vi "BASE.SaveConfig.vi"(8 "error in (no error)":errorcluster, 10 "config file path":path, 11 "Device.Simulation in":refnum<class "Device.Simulation.lvclass">) -> (0 "error out":errorcluster, 3 "Device.Simulation out":refnum<class "Device.Simulation.lvclass">)   [LabVIEW 2019, in "Device.Simulation.lvlib" / "Device.Simulation.lvclass"]
uses:
  Device.Simulation.lvclass
  Subsystems/BASE.Device/BASE.Device/BASE.Device.lvclass
  <vilib>/Utility/config.llb/NI_LVConfig.lvlib
panel:
  out "class name":string
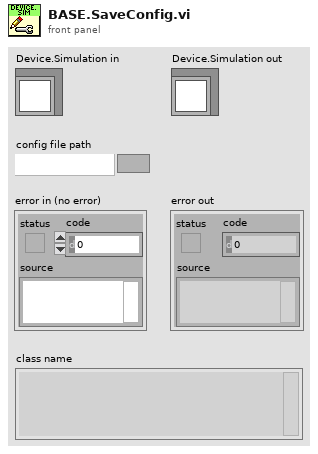
[diagram p1: front panel]
types:
  T1 = typedef "Device.Simulation.lvlib/Device.Simulation.lvclass/config--cluster.ctl" = cluster{"Name":string, "Time to Connect (ms)":u32, "Time to Check Connection (ms)":u32, "Time to Disconnect (ms)":u32, "Time to Read State (ms)":u32}
  T2 = typedef "NI_LVConfig.lvlib/Config Data RefNum.ctl" = refnum<k1>
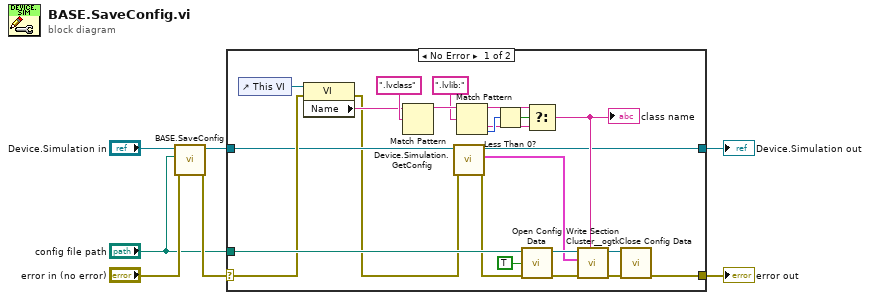
[diagram p0: block diagram]
diagram:
  n1 = call-parent "BASE.SaveConfig.vi"("error in (no error)"="error in (no error)", "config file path"="config file path", "BASE.Device in"="Device.Simulation in") -> ("error out"=w2:errorcluster, "BASE.Device out"=w5:refnum<class "Device.Simulation.lvclass">)  [unwired: 7 in]
  n2 = case shown="No Error" w2 {
    selector: w2 -> [w23 w32]
    tunnel: [w26 w32] -> w3
    tunnel: [w11 w31] -> w4
    tunnel: w5 -> [w12 w31]
    tunnel: "config file path" -> [w25 _]
    frame No Error {
      n3 = control-ref of="This VI"() -> (w24:refnum<vi>)
      n4 = property class="VI"(reference=w24, error in=w23) -> (error out=w10:errorcluster, "Name"=w14:string)  [unwired: 1 out]
      n5 = Match Pattern(string=w14, regular expression=".lvclass") -> (before substring=w20:string)  [unwired: 1 in, 3 out]
      n6 = call "Device.Simulation.GetConfig.vi"("error in (no error)"=w10, "Device.Simulation in"=w12) -> ("error out"=w9:errorcluster, "config"=w8:T1, "Device.Simulation out"=w11:refnum<class "Device.Simulation.lvclass">)  [unwired: 7 in]
      n7 = Match Pattern(string=w20, regular expression=".lvlib:") -> (before substring=w18:string, after substring=w17:string, offset past match=w21:i32)  [unwired: 1 in, 1 out]
      n8 = Less Than 0?(x=w21) -> (x < 0?=w19:bool)
      n9 = call <vilib>:"Open Config Data.vi"("error in (no error)"=w9, "create file if necessary (T)"=TRUE, "configuration file path"=w25) -> ("error out"=w29:errorcluster, "refnum"=w30:T2)  [unwired: 6 in, 1 out]
      n10 = Select(t=w18, s=w19, f=w17) -> (s? t:f=w13:string)
      "class name" <- w13
      n11 = call <userlib>:"Write Section Cluster__ogtk.vi"("section (optional)"=w13, "error in (no error)"=w29, "Section Formatted Cluster"=w8, "refnum"=w30) -> ("error out"=w28:errorcluster, "dup refnum"=w27:T2)  [unwired: 6 in]
      n12 = call <vilib>:"Close Config Data.vi"("error in (no error)"=w28, "refnum"=w27) -> ("error out"=w26:errorcluster)  [unwired: 8 in, 1 out]
    }
    frame Error {
    }
  }
  "error out" <- w3
  "Device.Simulation out" <- w4
